vi "Split number byte.vi"(5 "x":u8 format="%02x") -> (2 "lo(x)":u8 format="%02x", 3 "hi(x)":u8 format="%02x")   [LabVIEW 2013]
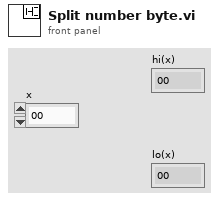
[diagram p1: front panel]
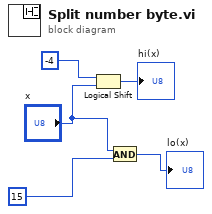
[diagram p0: block diagram]
diagram:
  n1 = Logical Shift(y=i16 -4, x="x") -> (x << y=→"hi(x)":u8)
  n2 = And(x="x", y=u8 15 ("and in")) -> (x .and. y?=→"lo(x)":u8)
